vi "GUI_laptop v9.vi"() -> ()   [LabVIEW 2019]
uses:
  <vilib>/Math Plots/3D Math Plots/3D Scatter/3D Scatter XCtrl/3D Scatter.xctl
  <vilib>/Platform/TimedLoop/XDataNode/timing_clust.ctl
  <vilib>/Platform/TimedLoop/XDataNode/nitl_modes.ctl
  <vilib>/Platform/TimedLoop/XDataNode/wakeup.ctl
  <vilib>/Analysis/_algsub.llb/Real Vector Norm.vi
  <vilib>/Instr/_visa.llb/VISA Configure Serial Port (Instr).vi
  <vilib>/Utility/file.llb/Write Delimited Spreadsheet (DBL).vi
  <vilib>/Math Plots/3D Math Plots/3D Scatter/3D Scatter Datatype/Public/Plot Helper (Vector).vi
  <vilib>/platform/TimedLoop/XDataNode/XDataNode.xnode
  <vilib>/Platform/TimedLoop/XDataNode/XDNodeRunTimeDep.lvlib
  <vilib>/Analysis/NI_AALPro.lvlib
  <vilib>/Math Plots/3D Math Plots/3D Scatter/3D Scatter Datatype/3D Scatter Datatype.lvclass
panel:
  in  "?":enum32{"Free Joystick", "Rigid Joystick"}(tab)
  in  "L1 bound (deg)":dbl=1000.0
  in  "L2 bound (deg)":dbl=1000.0
  in  "L3 bound (mm)":dbl=1000.0
  in  "L4 bound (deg)":dbl=1000.0
  in  "L5 bound":dbl=1000.0
  in  "y speed":dbl=0.5
  in  "z speed":dbl=0.5
  in  "x speed":dbl=0.5
  out "send values":dbl[](array[numeric])
  out "Robot Feedback (xyz)":dbl[](array[numeric])
  in  "UDP Send":bool
  in  "UDP Recv":bool
  in  "Joystick Type":dbl(ring) items=["Rigid Joystick", "Free Joystick"]
  out "Finished Late? [i-1]":bool
  in  "Epsilon":dbl=0.2
  out "3D Scatter":refnum<class "3D Plot Datatype.lvclass">[](xcontrol)
  out "Random Point":dbl[](array[numeric])
  out "Virtual Cursor":dbl[](array[numeric])
  out "Iteration Duration":i64
  in  "Num of Points":i32=10
  in  "z bound":dbl=2.0
  in  "y bound":dbl=5.0
  in  "x bound":dbl=5.0
  in  "Stop":bool
  in  "Round Decimals":dbl=2.0 format="%#_15g"
  in  "Save  Data":bool
  in  "Save Path":path
  out "error out":errorcluster
  in  "baud rate":u32=115200
  in  "VISA resource name":refnum<visa-resource-name>
  # "TODO: fix the bounds; currently bounds are arbitrary"
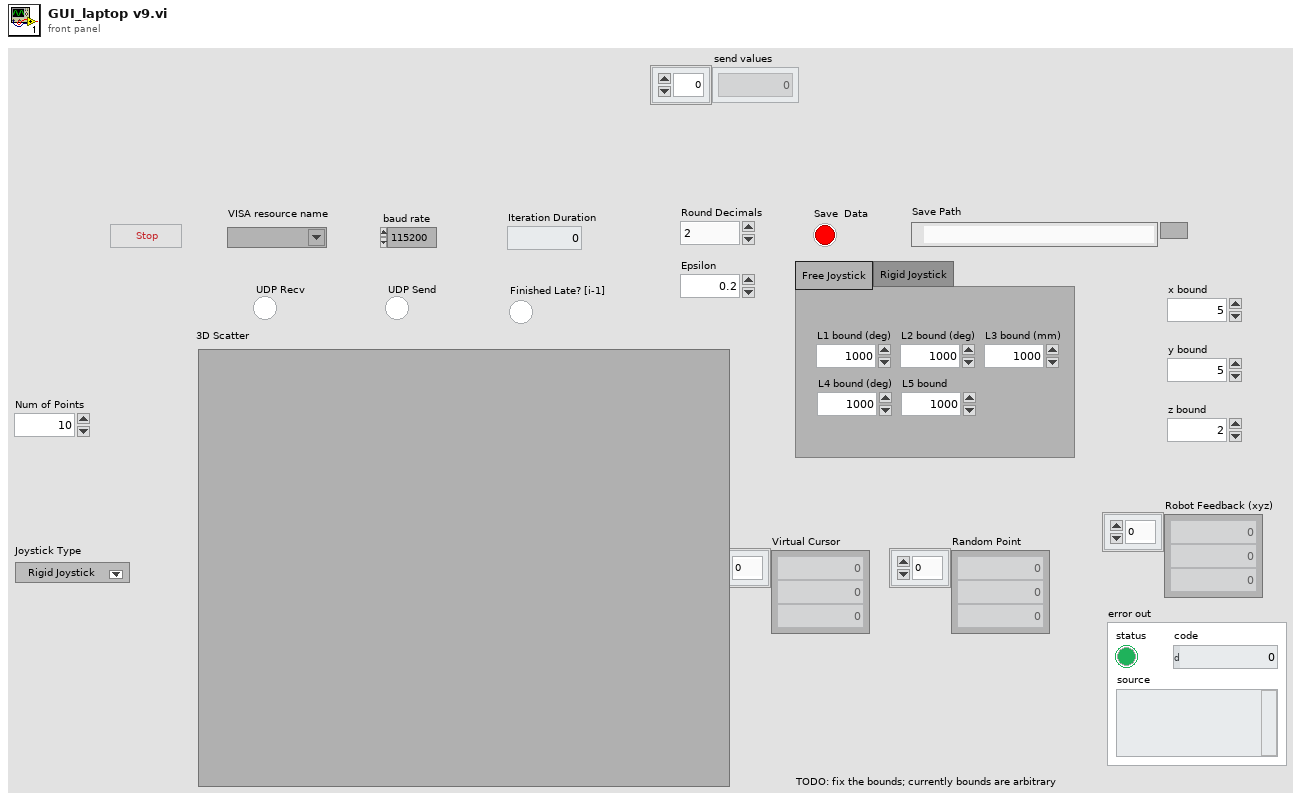
[diagram p1: front panel]
types:
  T1 = typedef "XDNodeRunTimeDep.lvlib/timing_clust.ctl" = cluster{"Expected End [f-1]":u64, "Actual End [f-1]":u64, "Finished Late? [f-1]":bool, "Expected End [i-1]":u64, "Actual End [i-1]":u64, "Finished Late? [i-1]":bool, "Expected Start [i]":u64, "Actual Start [i]":u64, "Expected Start [f]":u64, "Actual Start [f]":u64, "Source Name":string, "Structure Name":string, "Period":i64, "Deadline":i64, "Offset":i64, "Start":i64, "Priority":i32, "Timeout":i32, "Mode":T2, "Wakeup Reason":T3, "Error":errorcluster, "Source Type":string, "Secondary Source Type":string, "Global End Time":u64, "Global Start Time":u64, "Frame Duration":u64, "Iteration Duration":u64, "Assigned CPU":i32, "I/O Scan Engine Mode":u32}
  T2 = typedef "XDNodeRunTimeDep.lvlib/nitl_modes.ctl" = enum32{"No Change", "Process missed periods, maintain original phase", "Discard missed periods, maintain original phase", "Process missed periods, ignore original phase", "Discard missed periods, ignore original phase"}
  T3 = typedef "XDNodeRunTimeDep.lvlib/wakeup.ctl" = enum32{"Normal", "Aborted", "Asynchronous wakeup", "Timing source error", "Timed loop error", "Timeout"}
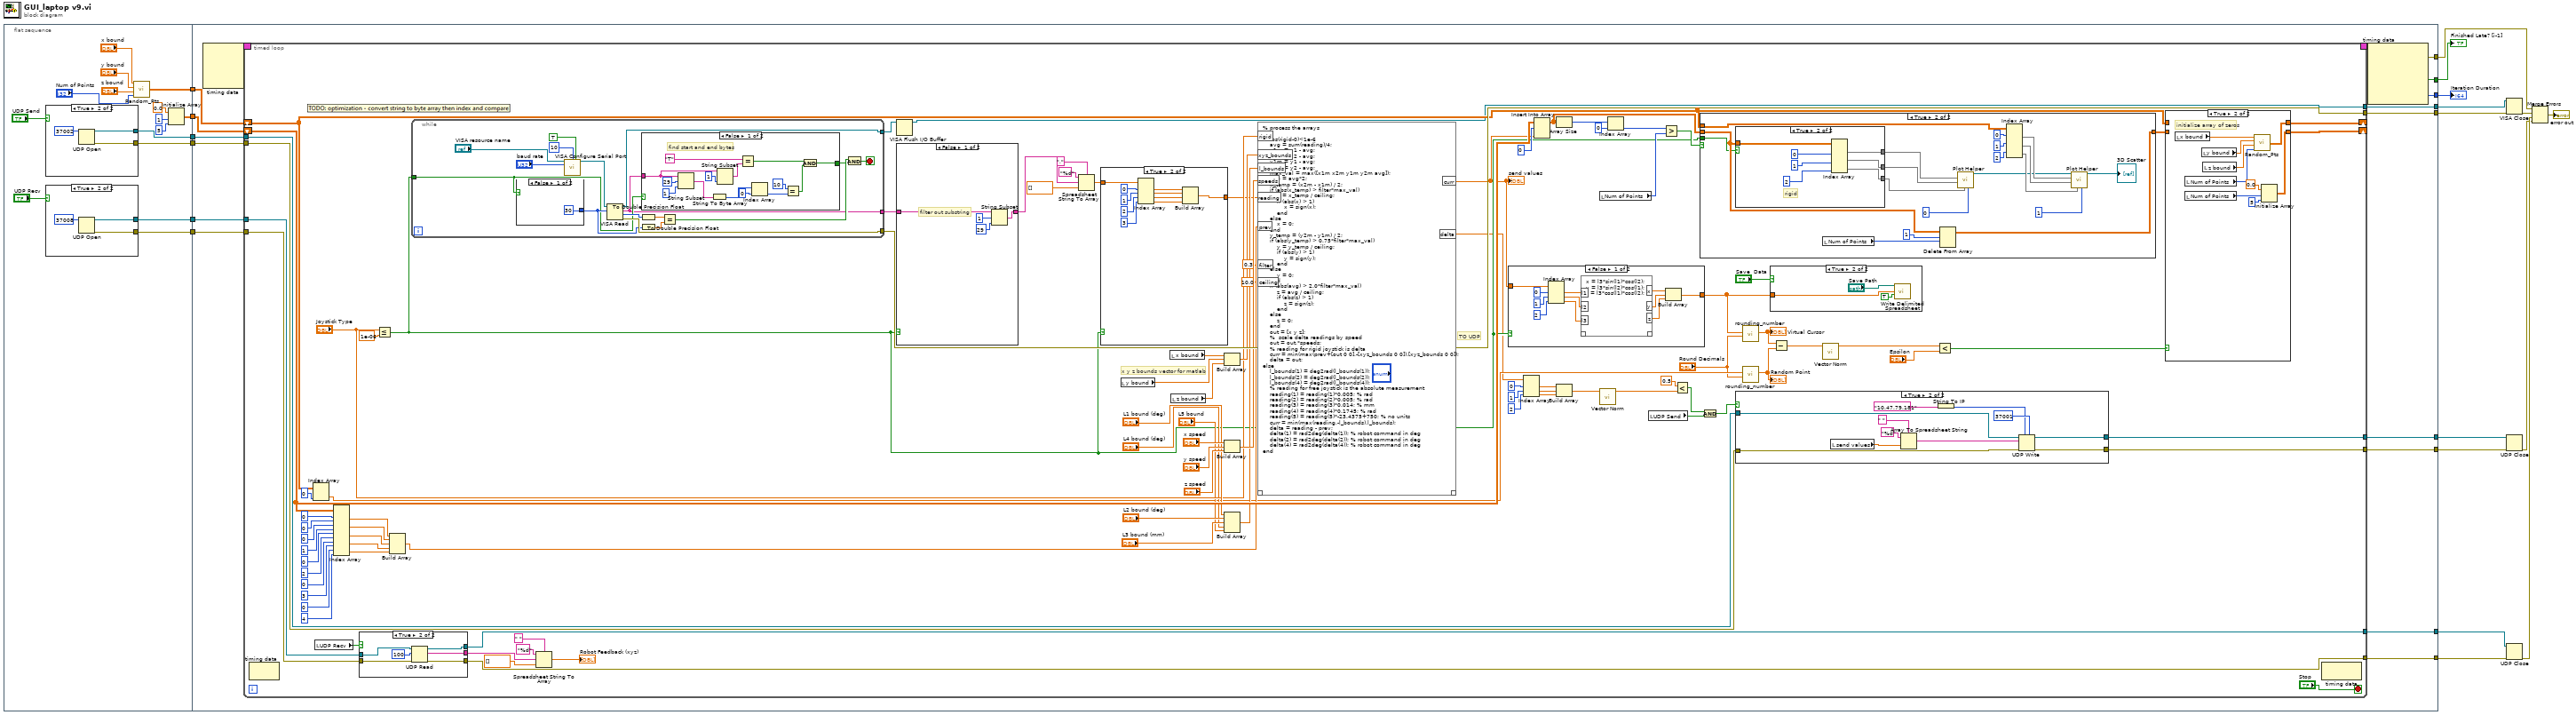
[diagram p0: block diagram]
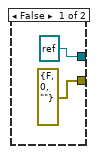
[diagram p2: hidden frame]
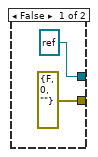
[diagram p3: hidden frame]
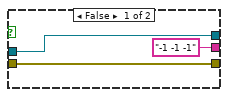
[diagram p5: hidden frame]
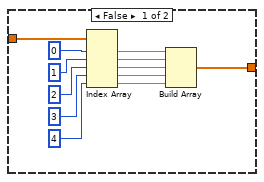
[diagram p9: hidden frame]
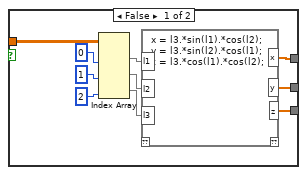
[diagram p12: hidden frame]
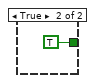
[diagram p13: hidden frame]
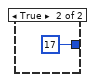
[diagram p14: hidden frame]
diagram:
  n1 = flat-sequence {
    tunnel: [w26] -> w15
    tunnel: [w30] -> w14
    tunnel: [w25] -> w13
    tunnel: [w24] -> w12
    tunnel: [w21] -> w11
    tunnel: [w20] -> w10
    tunnel: [w59] -> w19
    tunnel: [w58] -> w18
    tunnel: [w56] -> w9
    tunnel: [w54] -> w17
    tunnel: [w53] -> w16
    tunnel: w15 -> [w57]
    tunnel: w14 -> [w55]
    tunnel: w13 -> [w52]
    tunnel: w12 -> [w51]
    tunnel: w11 -> [w50]
    tunnel: w10 -> [w49]
    tunnel: [w48] -> w3
    tunnel: [w47] -> w8
    tunnel: [w46] -> w2
    tunnel: [w45] -> w1
    frame #0 {
      n2 = case shown="True" "UDP Send" {
        tunnel: [refnum<k16> refnum ("port") w38] -> w25
        tunnel: [errorcluster {"status"=FALSE, "code"=0, "source"=""} ("error out") w37] -> w20
        frame False {
        }
        frame True {
          n3 = UDP Open(11:u16 37002 ("port")) -> (port=w38:refnum<k16>, 0:w37:errorcluster)  [unwired: 4 in, 1 out]
        }
      }
      n4 = case shown="True" "UDP Recv" {
        tunnel: [refnum<k16> refnum ("port") w43] -> w24
        tunnel: [errorcluster {"status"=FALSE, "code"=0, "source"=""} ("error out") w42] -> w21
        frame False {
        }
        frame True {
          n5 = UDP Open(11:u16 37008 ("port")) -> (port=w43:refnum<k16>, 0:w42:errorcluster)  [unwired: 4 in, 1 out]
        }
      }
      n6 = call "Random_Pts.vi"("Num of Points"="Num of Points", "z bound"="z bound", "y bound"="y bound", "x bound"="x bound") -> ("appended array"=w30:dbl[][])
      n7 = Initialize Array(0.0 ("element"), 1 ("dimension size"), 5 ("dimension size")) -> (w26:dbl[][])
    }
    frame #1 {
      n8 = node-c288() -> (w61:T1)  [unwired: 4 in]
      n9 = timed-loop {
        tunnel: [w92] -> w59
        tunnel: [w157] -> w58
        shift-right: [w156] -> _
        shift-left: w57 -> [w155]
        timing: w61 -> [_]
        timing-out: [_] -> w60
        shift-right: [w151] -> _
        shift-left: w55 -> [w152]
        tunnel: w52 -> [w91]
        tunnel: w51 -> [w90]
        tunnel: w50 -> [w88]
        tunnel: w49 -> [w87]
        tunnel: [w86] -> w48
        tunnel: [w85] -> w47
        tunnel: [w84] -> w46
        tunnel: [w83] -> w45
        stop <- "Stop" stop-if-true
        # "TO UDP"
        # "MATLAB IS ROW VECTOR"
        # "x y z bounds vector for matlab"
        n10 = node-c288() -> ()  [unwired: 1 in, 1 out]
        n11 = Index Array(array=w152, index (col)=0 ("index (row)")) -> (element=w103:dbl[])  [unwired: 1 in]
        n12 = local read "UDP Recv"() -> (w89:bool)
        n13 = Index Array(array=w155, index (row) #1=0 ("disabled index (row)"), index (col) #1=0 ("disabled index (col)"), index (row) #2=0 ("disabled index (row)"), index (col) #2=1 ("disabled index (col)"), index (row) #3=0 ("disabled index (row)"), index (col) #3=2 ("disabled index (col)"), index (row) #4=0 ("disabled index (row)"), index (col) #4=3 ("disabled index (col)"), index (row) #5=0 ("disabled index (row)"), index (col) #5=4 ("disabled index (col)")) -> (element #1=w128:dbl, element #2=w127:dbl, element #3=w126:dbl, element #4=w112:dbl, element #5=w111:dbl)
        n14 = case shown="True" w89 {
          tunnel: w90 -> [w173 w180]
          tunnel: w88 -> [w174 w179]
          tunnel: [w174 w178] -> w86
          tunnel: [w173 w177] -> w84
          tunnel: ["-1 -1 -1" w175] -> w79
          frame False {
          }
          frame True {
            n15 = UDP Read(connection ID=w180, max size (548)=100, 8:w179) -> (data out=w175:string, error out=w178:errorcluster, 3:w177:refnum<k16>)  [unwired: 1 in, 2 out]
          }
        }
        n16 = Less Or Equal?(x="Joystick Type", y=1e-06) -> (x <= y?=w105:bool)
        n17 = Build Array(w128, w127, w126, w112, w111) -> (w125:dbl[])
        n18 = while {
          tunnel: [w271] -> w106
          tunnel: [w284] -> w157
          tunnel: [w278] -> w93
          tunnel: w105 -> [w272]
          stop <- w274 stop-if-true
          n19 = case shown="False" w272 {
            tunnel: [30 u32 17 ("byte count")] -> w277
            frame False {
            }
            frame True {
            }
          }
          n20 = call-poly "VISA Configure Serial Port"("VISA resource name"="VISA resource name", "termination char\n(0xA = '\\n' = LF)"=u8 10 ("termination char\n(0xA = '\\n' = LF)"), "Enable Termination\nChar (T)"=TRUE ("Enable Termination\nChar (T)"), "baud rate (9600)"="baud rate") -> ("VISA resource name out"=w279:refnum<visa-resource-name>)  [unwired: 10 in, 1 out]
          n21 = VISA Read(VISA resource name=w279, byte count=w277) -> (VISA resource name out=w278:refnum<visa-resource-name>, read buffer=w271:string, return count=w286:u32, error out=w284:errorcluster)  [unwired: 1 in]
          n22 = To Double Precision Float(number=w286) -> (double precision float=w285:dbl)
          n23 = To Double Precision Float(number=w277) -> (double precision float=w276:dbl)
          n24 = case shown="False" w272 {
            tunnel: [w293 TRUE] -> w273
            tunnel: w271 -> [w296 _]
            frame False {
              # "find start and end bytes"
              n25 = String Subset(string=w296, offset (0)=29, length (rest)=1) -> (substring=w291:string)
              n26 = String To Byte Array(string=w291) -> (unsigned byte array=w290:u8[])
              n27 = String Subset(string=w296, length (rest)=1) -> (substring=w299:string)  [unwired: 1 in]
              n28 = Equal?(x="T", y=w299) -> (x = y?=w295:bool)
              n29 = Index Array(array=w290, index=0) -> (element=w288:u8)
              n30 = Equal?(x=10, y=w288) -> (x = y?=w294:bool)
              n31 = And(x=w295, y=w294) -> (x .and. y?=w293:bool)
            }
            frame True {
            }
          }
          n32 = Equal?(x=w285, y=w276) -> (x = y?=w275:bool)
          n33 = And(x=w275, y=w273) -> (x .and. y?=w274:bool)
        }
        n34 = Spreadsheet String To Array(delimiter (Tab)=" ", format string="%d", spreadsheet string=w79, array type (2D Dbl)=dbl[] []) -> (array=→"Robot Feedback (xyz)":dbl[])
        n35 = VISA Flush I/O Buffer(VISA resource name=w93) -> (VISA resource name out=w92:refnum<visa-resource-name>)  [unwired: 2 in, 1 out]
        n36 = case shown="False" w105 {
          tunnel: w106 -> [w198 w199]
          tunnel: [w195 w199] -> w104
          frame False {
            # "filter out substring"
            n37 = String Subset(string=w198, offset (0)=1, length (rest)=29) -> (substring=w195:string)
          }
          frame True {
          }
        }
        n38 = Spreadsheet String To Array(delimiter (Tab)=",", format string="%d", spreadsheet string=w104, array type (2D Dbl)=dbl[] []) -> (array=w108:dbl[])
        n39 = case shown="True" w105 {
          tunnel: w108 -> [w200 w215]
          tunnel: [w205 w214] -> w107
          frame False {
            n40 = Index Array(array=w200, index #1=0 ("Plot ID"), index #2=1 ("Plot ID"), index #3=2 ("Plot ID"), index #4=3 ("Plot ID"), index #5=4 ("Plot ID")) -> (element #1=w208:dbl, element #2=w207:dbl, element #3=w206:dbl, element #4=w202:dbl, element #5=w201:dbl)
            n41 = Build Array(w208, w207, w206, w202, w201) -> (w205:dbl[])
          }
          frame True {
            n42 = Index Array(array=w215, index #1=0 ("Plot ID"), index #2=1 ("Plot ID"), index #3=2 ("Plot ID"), index #4=3 ("index")) -> (element #1=w218:dbl, element #2=w217:dbl, element #3=w216:dbl, element #4=w212:dbl)
            n43 = Build Array(w218, w217, w216, w212) -> (w214:dbl[])
          }
        }
        n44 = local read "y bound"() -> (w130:dbl)
        n45 = local read "x bound"() -> (w131:dbl)
        n46 = local read "z bound"() -> (w129:dbl)
        n47 = Build Array(w131, w130, w129) -> (w123:dbl[])
        n48 = Build Array("x speed", "y speed", "z speed") -> (w124:dbl[])
        n49 = Build Array("L1 bound (deg)", "L2 bound (deg)", "L3 bound (mm)", "L4 bound (deg)", "L5 bound") -> (w119:dbl[])
        n50 = script code="% process the arrays\n\nif abs(rigid-0)<1e-6\n    avg = sum(reading)/4;\n    x1m = x1 - avg;\n    x2m = x2 - avg;\n    y1m = y1 - avg;\n    y2m = y2 - avg;\n    max_val = max([x1m x2m y1m y2m avg]);\n    avg = avg*2;\n    x_temp = (x2m - x1m) / 2;\n    if (abs(x_temp) > filter*max_val)\n        x = x_temp / ceiling;\n        if (abs(x) > 1)\n            x = sign(x);\n        end\n    else\n        x = 0;\n    end\n    y_temp = (y2m - y1m) / 2;\n    if (abs(y_temp) > 0.75*filter*max_val)\n        y = y_temp / ceiling;\n        if (abs(y) > 1)\n            y = sign(y);\n        end\n    else\n        y = 0;\n    end\n    if (abs(avg) > 2.0*filter*max_val)\n        z = avg / ceiling;\n        if (abs(z) > 1)\n            z = sign(z);\n        end\n    else\n        z = 0;\n    end\n    out = [x y z];\n    %  scale delta readings by speed\n    out = out.*speeds;\n    % reading for rigid joystick is delta\n    curr = min(max(prev+[out 0 0],-[xyz_bounds 0 0]),[xyz_bounds 0 0]);\n    delta = out;\nelse\n    l_bounds(1) = deg2rad(l_bounds(1));\n    l_bounds(2) = deg2rad(l_bounds(2));\n    l_bounds(4) = deg2rad(l_bounds(4));\n    % reading for free joystick is the absolute measurement\n    reading(1) = reading(1)*0.005; % rad\n    reading(2) = reading(2)*0.005; % rad\n    reading(3) = reading(3)*0.014; % mm\n    reading(4) = reading(4)*0.1745; % rad\n    reading(5) = reading(5)*-23.4375+750; % no units\n    curr = min(max(reading,-l_bounds),l_bounds);\n    delta = reading - prev;\n    delta(1) = rad2deg(delta(1)); % robot command in deg\n    delta(2) = rad2deg(delta(2)); % robot command in deg\n    delta(4) = rad2deg(delta(4)); % robot command in deg\nend"("xyz_bounds"=w123, "speeds"=w124, "reading"=w107, "prev"=w125, "rigid"="Joystick Type", "l_bounds"=w119, "ceiling"=10.0 ("Real"), "filter"=0.3 ("Real")) -> ("curr"=w64:dbl[], "delta"=w72:dbl[])  [unwired: 1 in, 1 out]
        "send values" <- w64
        n51 = case shown="False" w105 {
          tunnel: w64 -> [w229 w233]
          tunnel: [w222 w233] -> w153
          frame False {
            n52 = Index Array(array=w229, index #1=0 ("Plot ID"), index #2=1 ("Plot ID"), index #3=2 ("Plot ID")) -> (element #1=w228:dbl, element #2=w227:dbl, element #3=w226:dbl)
            n53 = script code="x = l3*sin(l1)*cos(l2);\ny = l3*sin(l2)*cos(l1);\nz = l3*cos(l1)*cos(l2);"("l1"=w228, "l2"=w227, "l3"=w226) -> ("x"=w225:dbl, "y"=w224:dbl, "z"=w223:dbl)  [unwired: 1 in, 1 out]
            n54 = Build Array(w225, w224, w223) -> (w222:dbl[])
          }
          frame True {
          }
        }
        n55 = Index Array(array=w72, index #1=0 ("disabled index (col)"), index #2=1 ("disabled index (col)"), index #3=2 ("disabled index (col)")) -> (element #1=w68:dbl, element #2=w67:dbl, element #3=w66:dbl)
        n56 = Insert Into Array(array=w155, index (row)=0, new element=w64) -> (w136:dbl[][])  [unwired: 1 in]
        n57 = Array Size(array=w136) -> (size(s)=w138:i32[])
        n58 = Build Array(w68, w67, w66) -> (w65:dbl[])
        n59 = local read "Num of Points"() -> (w137:i32)
        n60 = call-poly <vilib>:"Vector Norm.vi"("Input Vector"=w65) -> ("norm"=w77:dbl)  [unwired: 9 in, 1 out]
        n61 = Index Array(array=w138, index=0) -> (element=w139:i32)
        n62 = local read "UDP Send"() -> (w74:bool)
        n63 = Greater?(x=w139, y=w137) -> (0:w135:bool)
        n64 = Less?(x=0.5, y=w77) -> (x < y?=w75:bool)
        n65 = case shown="True" w135 {
          tunnel: w136 -> [w234 w252]
          tunnel: [w234 w251] -> w154
          tunnel: w152 -> [_ w250]
          tunnel: w105 -> [_ w235]
          frame False {
          }
          frame True {
            n66 = case shown="True" w235 {
              tunnel: w252 -> [w263 w267]
              tunnel: [w254 w266] -> w241
              tunnel: [w255 w265] -> w240
              tunnel: [w256 w264] -> w239
              frame False {
                n67 = Index Array(array=w263, index (col) #1=0 ("Plot ID"), index (col) #2=1 ("Plot ID"), index (col) #3=2 ("Plot ID")) -> (element #1=w259:dbl[], element #2=w258:dbl[], element #3=w257:dbl[])  [unwired: 3 in]
                n68 = script code="x = l3.*sin(l1).*cos(l2);\ny = l3.*sin(l2).*cos(l1);\nz = l3.*cos(l1).*cos(l2);"("l1"=w259, "l2"=w258, "l3"=w257) -> ("x"=w254:dbl[], "y"=w255:dbl[], "z"=w256:dbl[])  [unwired: 1 in, 1 out]
              }
              frame True {
                # "rigid"
                n69 = Index Array(array=w267, index (col) #1=0 ("disabled index (col)"), index (col) #2=1 ("index (col)"), index (col) #3=2 ("index (col)")) -> (element #1=w266:dbl[], element #2=w265:dbl[], element #3=w264:dbl[])  [unwired: 3 in]
              }
            }
            n70 = local read "Num of Points"() -> (w249:i32)
            n71 = Delete From Array(array=w252, length=1, index (row)=w249) -> (array with subset deleted=w251:dbl[][])  [unwired: 1 in, 1 out]
            n72 = call-poly <vilib>:"Plot Helper.vi"("Plot ID"=0, "z vector"=w239, "y vector"=w240, "x vector"=w241) -> ("3D Plot lvclass Array out"=w243:refnum<class "3D Plot Datatype.lvclass">[])  [unwired: 2 in, 5 out]
            n73 = Index Array(array=w250, index (row) #1=0 ("index (row)"), index (row) #2=1 ("index (row)"), index (row) #3=2 ("index (row)")) -> (element #1=w247:dbl[], element #2=w246:dbl[], element #3=w245:dbl[])  [unwired: 3 in]
            n74 = call-poly <vilib>:"Plot Helper.vi"("Plot ID"=1, "z vector"=w245, "y vector"=w246, "x vector"=w247, "3D Plot lvclass Array in"=w243) -> ("3D Plot lvclass Array out"=→"3D Scatter":refnum<class "3D Plot Datatype.lvclass">[])  [unwired: 1 in, 5 out]
          }
        }
        n75 = And(x=w75, y=w74) -> (x .and. y?=w73:bool)
        n76 = case shown="True" w73 {
          tunnel: w91 -> [w159 w171]
          tunnel: w87 -> [w160 w167]
          tunnel: [w160 w163] -> w85
          tunnel: [w159 w162] -> w83
          frame False {
          }
          frame True {
            n77 = local read "send values"() -> (w161:dbl[])
            n78 = Array To Spreadsheet String(delimiter (Tab)=" ", array=w161, 3:"%d" ("format string")) -> (spreadsheet string=w168:string)
            n79 = String To IP(1:"10.47.79.181" ("name")) -> (0:w165:u32)
            n80 = UDP Write(address=w165, port or service name=u16 37001, connection ID=w171, data in=w168, 8:w167) -> (error out=w163:errorcluster, 3:w162:refnum<k16>)  [unwired: 1 in]
          }
        }
        n81 = call "rounding_number.vi"("power of ten"="Round Decimals", "Array"=w153) -> ("rounded"=w100:dbl[])  [unwired: 9 in]
        "Virtual Cursor" <- w100
        n82 = call "rounding_number.vi"("power of ten"="Round Decimals", "Array"=w103) -> ("rounded"=w99:dbl[])  [unwired: 9 in]
        "Random Point" <- w99
        n83 = case shown="True" "Save  Data" {
          tunnel: w153 -> [_ w181]
          frame False {
          }
          frame True {
            n84 = call-poly <vilib>:"Write Delimited Spreadsheet.vi"("file path (dialog if empty)"="Save Path", "1D data"=w181, "append to file? (new file:F)"=TRUE) -> ()  [unwired: 11 in, 2 out]
          }
        }
        n85 = Subtract(x=w100, y=w99) -> (x-y=w98:dbl[])
        n86 = call-poly <vilib>:"Vector Norm.vi"("Input Vector"=w98) -> ("norm"=w97:dbl)  [unwired: 9 in, 1 out]
        n87 = Less?(x=w97, y="Epsilon") -> (x < y?=w95:bool)
        n88 = case shown="True" w95 {
          tunnel: w152 -> [w185 _]
          tunnel: [w185 w190] -> w151
          tunnel: w154 -> [w184 _]
          tunnel: [w184 w186] -> w156
          frame False {
          }
          frame True {
            # "initialize array of zeros"
            n89 = local read "x bound"() -> (w194:dbl)
            n90 = local read "Num of Points"() -> (w191:i32)
            n91 = local read "Num of Points"() -> (w188:i32)
            n92 = local read "y bound"() -> (w193:dbl)
            n93 = local read "z bound"() -> (w192:dbl)
            n94 = call "Random_Pts.vi"("Num of Points"=w191, "z bound"=w192, "y bound"=w193, "x bound"=w194) -> ("appended array"=w190:dbl[][])
            n95 = Initialize Array(0.0 ("element"), w188, 5 ("dimension size")) -> (w186:dbl[][])
          }
        }
        n96 = node-c288() -> ()  [unwired: 1 in, 1 out]
      }
      n97 = node-c288(w60) -> (w56:errorcluster, w53:bool, w54:i64)  [unwired: 3 out]
    }
  }
  n98 = VISA Close(VISA resource name=w19, error in (no error)=w18) -> (error out=w7:errorcluster)
  n99 = UDP Close(connection ID=w1, 8:w8) -> (error out=w5:errorcluster)  [unwired: 1 out]
  n100 = UDP Close(connection ID=w2, 8:w3) -> (error out=w6:errorcluster)  [unwired: 1 out]
  n101 = Merge Errors(w9, w7, w6, w5) -> (→"error out":errorcluster)
  "Iteration Duration" <- w17
  "Finished Late? [i-1]" <- w16
